vi "Add Projection Keys.vi"(10 "Projection Info":T1[](array[typedef]), 11 "Class Ref Map":variant) -> (3 "Augmented Class Ref Map":variant)   [LabVIEW 2013]
uses:
  Data Structures/JSON/Projection Info.ctl
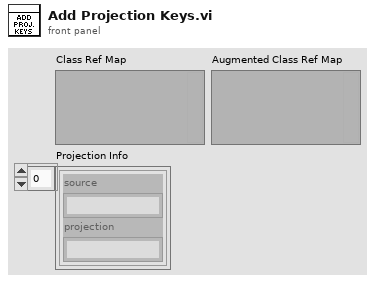
[diagram p1: front panel]
types:
  T1 = typedef "Projection Info.ctl" = cluster{"source":string, "projection":string}
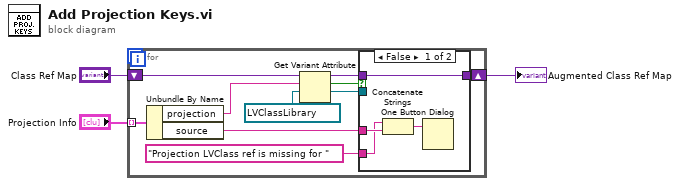
[diagram p0: block diagram]
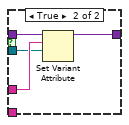
[diagram p2: hidden frame]
diagram:
  n1 = for {
    tunnel: "Projection Info" -> [w13] mode=indexing
    shift-right: [w7] -> w1
    shift-left: "Class Ref Map" -> [w12]
    n2 = Unbundle By Name(w13) -> ("projection"=w11:string, "source"=w6:string)
    n3 = Get Variant Attribute(Variant=w12, name=w11, default value (empty Variant)=refnum<vi> refnum ("Object Ref")) -> (duplicate Variant=w8:variant, found=w9:bool, value=w5:refnum<vi>)  [unwired: 1 in, 1 out]
    n4 = case shown="False" w9 {
      tunnel: w8 -> [w17 w21]
      tunnel: [w17 w20] -> w7
      tunnel: w6 -> [w16 w19]
      tunnel: w5 -> [_ w18]
      tunnel: "Projection LVClass ref is missing for " -> [w14 _]
      frame False {
        n5 = Concatenate Strings(w14, w16) -> (w15:string)
        n6 = One Button Dialog(message=w15) -> ()  [unwired: 1 in, 1 out]
      }
      frame True {
        n7 = Set Variant Attribute(Variant=w21, name=w19, value=w18) -> (Variant out=w20:variant)  [unwired: 1 in, 2 out]
      }
    }
  }
  "Augmented Class Ref Map" <- w1
